vi "pic_JudgeMotionALL.vi"(3 "error in)":errorcluster, 4 "Limit":bool[](array[boolean]), 5 "CmdLib In":refnum<k24>) -> (0 "error out":errorcluster, 2 "CmdLib Out":refnum<k24>)   [LabVIEW 2018]
uses:
  Device VIs/CmdLib.dll
  Device VIs/Verbal.vi
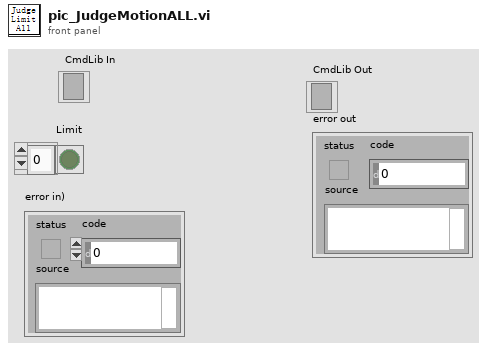
[diagram p1: front panel]
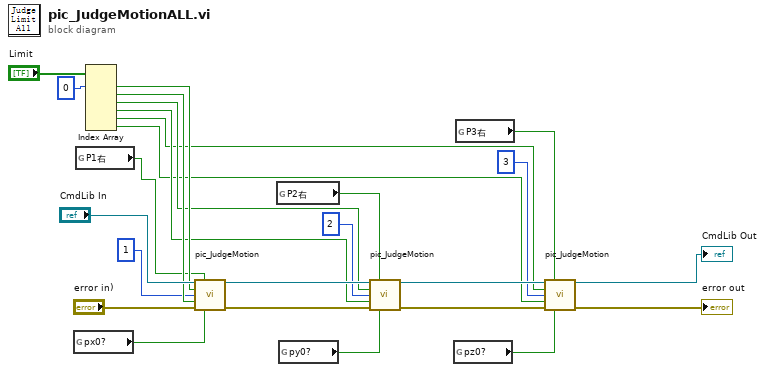
[diagram p0: block diagram]
diagram:
  n1 = global read "Verbal.vi" "px0?"() -> (w17:bool)
  n2 = global read "Verbal.vi" "P1右"() -> (w18:bool)
  n3 = Index Array(array="Limit", index #1=0 ("索引")) -> (element #1=w21:bool, element #2=w20:bool, element #3=w14:bool, element #4=w13:bool, element #5=w7:bool, element #6=w6:bool)  [unwired: 5 in]
  n4 = call "pic_JudgeMotion.vi"("CmdLib In"="CmdLib In", "右？"=w18, "Llimit"=w21, "Motor"=1, "Rlimit"=w20, "error in (no error)"="error in)", "零位？"=w17) -> ("CmdLib Out"=w16:refnum<k24>, "error out"=w15:errorcluster)  [unwired: 7 in]
  n5 = global read "Verbal.vi" "P2右"() -> (w10:bool)
  n6 = global read "Verbal.vi" "py0?"() -> (w11:bool)
  n7 = call "pic_JudgeMotion.vi"("CmdLib In"=w16, "右？"=w10, "Llimit"=w14, "Motor"=2, "Rlimit"=w13, "error in (no error)"=w15, "零位？"=w11) -> ("CmdLib Out"=w9:refnum<k24>, "error out"=w8:errorcluster)  [unwired: 7 in]
  n8 = global read "Verbal.vi" "pz0?"() -> (w3:bool)
  n9 = global read "Verbal.vi" "P3右"() -> (w4:bool)
  n10 = call "pic_JudgeMotion.vi"("CmdLib In"=w9, "右？"=w4, "Llimit"=w7, "Motor"=3, "Rlimit"=w6, "error in (no error)"=w8, "零位？"=w3) -> ("CmdLib Out"=→"CmdLib Out":refnum<k24>, "error out"=→"error out":errorcluster)  [unwired: 7 in]
